vi "Remote1Joystick2.vi"() -> (18 "X Axis":i8, 19 "Y Axis":i8)   [LabVIEW 2012, in "FTC.lvlib" / "Remote Interface.lvlib"]
uses:
  Remote Interface.lvlib
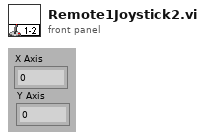
[diagram p1: front panel]
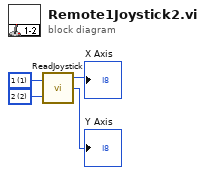
[diagram p0: block diagram]
diagram:
  w3 = u8 2 items=["1"=1, "2"=2] ("Joystick Number (1)")
  w4 = u8 1 items=["1"=1, "2"=2] ("Remote (1)")
  n1 = call "ReadJoystick.vi"("Joystick Number (1)"=w3, "Remote (1)"=w4) -> ("Y Axis"=→"Y Axis":i8, "X Axis"=→"X Axis":i8)  [unwired: 1 out]
